vi "dfd_Render Real and Complex Roots+.vi"(0 "variable":string="z", 1 "alignment(left, top)":T3, 4 "display format":T2 items=["Separated Roots", "Combined Roots"], 5 "format coeffiecients":string, 6 "bracket":cluster{"left":string, "right":string}={"left"="(", "right"=")"}, 7 "fonts input":T5(array[cluster]), 8 "format control":T1={"display \"1\" when there are no roots"=TRUE, "bracket force to add"=FALSE}, 9 "origin":cluster{"x":i16, "y":i16}, 10 "Roots":cdb[](array[numeric]), 11 "picture in":picture) -> (2 "total rect":T4, 3 "picture out":picture)   [LabVIEW 2017, in "NI_DigFilter_Process.lvlib"]
uses:
  <vilib>/addons/Digital Filter Design/NI_DigFilter_Process.lvlib
  <vilib>/addons/Digital Filter Design/Render.llb/dfd_ZPK Display Format.ctl
  <vilib>/Analysis/NI_AALPro.lvlib
panel:
  in  "Tolerance for real roots":dbl
  in  "Tolerance for conjugate pair":dbl
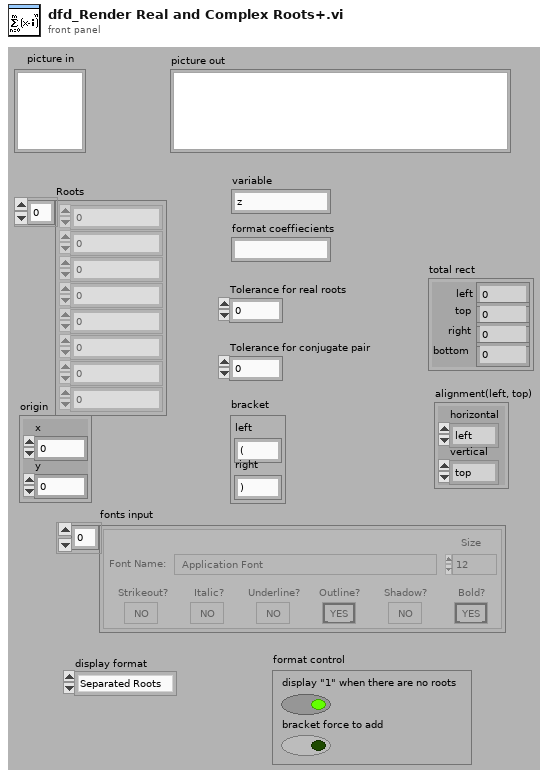
[diagram p1: front panel]
types:
  T1 = cluster{"display \"1\" when there are no roots":bool, "bracket force to add":bool}
  T2 = typedef "dfd_ZPK Display Format.ctl" = u16
  T3 = cluster{"horizontal":enum16{"left", "center", "right"}, "vertical":enum16{"top", "center", "bottom"}}
  T4 = cluster{"left":i16, "top":i16, "right":i16, "bottom":i16}
  T5 = cluster{"Font Name:":string, "Size":i16, "Strikeout?":bool, "Italic?":bool, "Underline?":bool, "Outline?":bool, "Shadow?":bool, "Bold?":bool}[]
  T6 = enum16{"User-specified Font", "Application Font", "System Font", "Dialog Font"}
  T7 = cluster{"Font Name:":string, "Size":i16, "Strikeout?":bool, "Italic?":bool, "Underline?":bool, "Outline?":bool, "Shadow?":bool, "Bold?":bool}
  T8 = typedef "imagedata.ctl" = cluster{"image type":i32, "image depth":i32, "image":u8[], "mask":u8[], "colors":u32[], "Rectangle":cluster{"left":i16, "top":i16, "right":i16, "bottom":i16}}
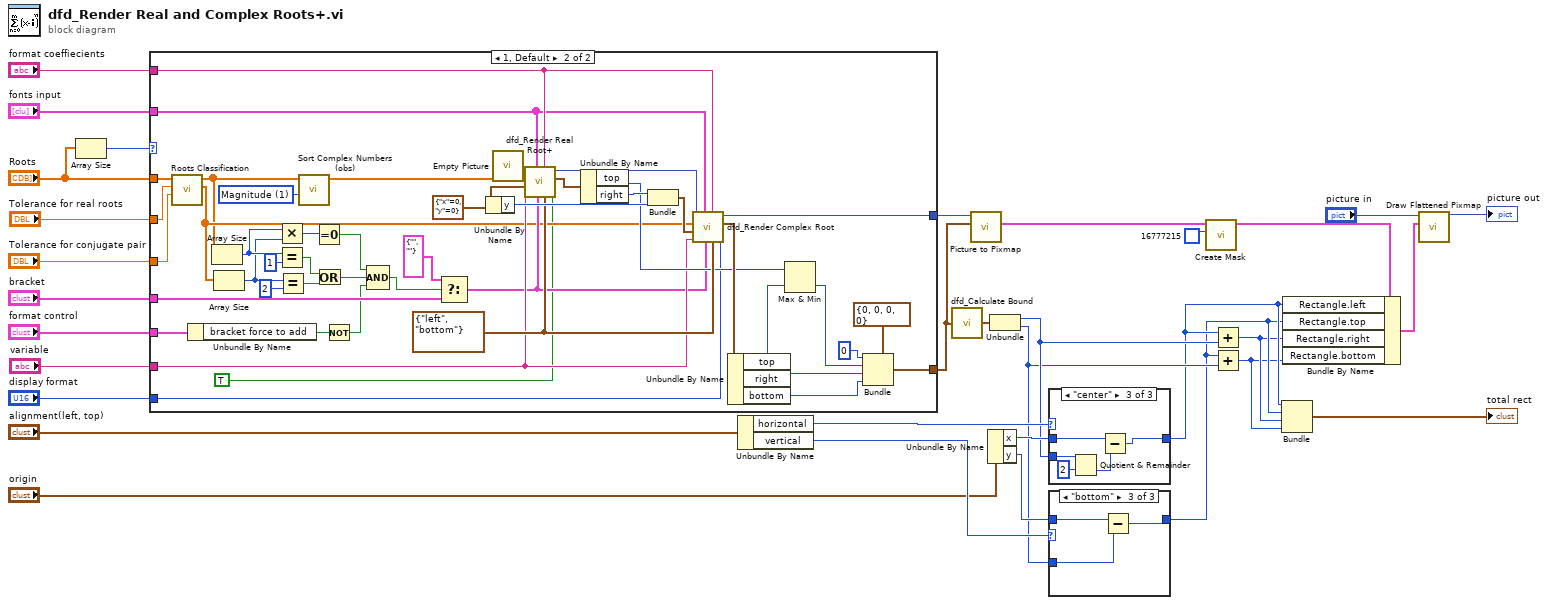
[diagram p0: block diagram]
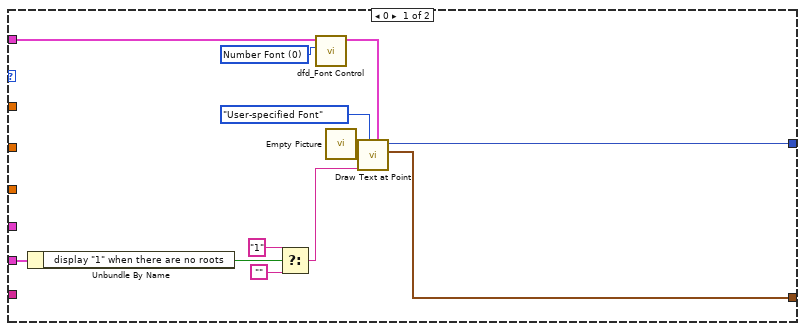
[diagram p2: hidden frame]
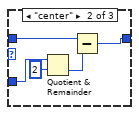
[diagram p4: hidden frame]
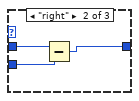
[diagram p6: hidden frame]
diagram:
  n1 = Array Size(array="Roots") -> (size(s)=w2:i32)
  n2 = case shown="1, Default" w2 {
    tunnel: "Tolerance for conjugate pair" -> [_ w90]
    tunnel: "Tolerance for real roots" -> [_ w89]
    tunnel: [w43 w83] -> w30
    tunnel: [w44 w77] -> w23
    tunnel: "format coeffiecients" -> [_ w69]
    tunnel: "fonts input" -> [w41 w68]
    tunnel: "display format" -> [_ w45]
    tunnel: "variable" -> [_ w66]
    tunnel: "Roots" -> [_ w65]
    tunnel: "bracket" -> [_ w62]
    tunnel: "format control" -> [w34 w49]
    frame 0 {
      w39 = u16 0 items=["Number Font", "Variable Font", "Script Font"] ("Tpye")
      n3 = Unbundle By Name(w34) -> ("display \"1\" when there are no roots"=w33:bool)
      n4 = Select(t="1" ("text"), s=w33, f="") -> (s? t:f=w36:string)
      n5 = call <vilib>:"dfd_Font Control.vi"("tpye"=w39, "fonts input"=w41) -> ("font output"=w40:T7)  [unwired: 9 out]
      n6 = call "Empty Picture"() -> ("empty picture"=w38:picture)
      n7 = call <vilib>:"Draw Text at Point.vi"("[user-specified font]"=w40, "desired font(Application)"=T6."User-specified Font", "text"=w36, "picture"=w38) -> ("text rect"=w44:T4, "new picture"=w43:picture)  [unwired: 5 in, 1 out]
    }
    frame 1, Default {
      w74 = cluster{"x":i16, "y":i16} {"x"=0, "y"=0} ("origin")
      w76 = T3 {"horizontal"=enum."left", "vertical"=enum."bottom"} ("alignment(left, top)")
      w88 = u16 1 items=["Real & Imaginary", "Magnitude"] ("method")
      n8 = call <vilib>:"Roots Classification.vi"("tolerance for conjugate pair"=w90, "tolerance for real roots"=w89, "Roots"=w65) -> ("Complex Pair Roots"=w60:cdb[], "Real Roots"=w58:dbl[])  [unwired: 7 out]
      n9 = Unbundle By Name(w49) -> ("bracket force to add"=w48:bool)
      n10 = Array Size(array=w58) -> (size(s)=w57:i32)
      n11 = Array Size(array=w60) -> (size(s)=w56:i32)
      n12 = Multiply(x=w57, y=w56) -> (x*y=w55:i32)
      n13 = Equal?(x=w57, y=1) -> (x = y?=w54:bool)
      n14 = Equal?(x=w56, y=2) -> (x = y?=w53:bool)
      n15 = call <vilib>:"Sort Complex Numbers (obs).vi"("method"=w88, "Complex Numbers"=w58) -> ("Sorted Complex Numbers"=w67:cdb[])  [unwired: 1 in, 8 out]
      n16 = Equal To 0?(x=w55) -> (x = 0?=w51:bool)
      n17 = Or(x=w54, y=w53) -> (x .or. y?=w52:bool)
      n18 = Not(x=w48) -> (.not. x?=w47:bool)
      n19 = Compound Arithmetic op=AND(w51, w52, w47) -> (w50:bool)
      n20 = Select(t=cluster{"left":string, "right":string} {"left"="", "right"=""} ("bracket"), s=w50, f=w62) -> (s? t:f=w61:cluster{"left":string, "right":string})
      n21 = Unbundle By Name(w74) -> ("y"=w78:i16)
      n22 = call "Empty Picture"() -> ("empty picture"=w73:picture)
      n23 = call <vilib>:"dfd_Render Real Root+.vi"("Negative Exponent?"=TRUE ("negative exponent? 2"), "alignment(left, top)"=w76, "format string"=w69, "bracket"=w61, "Fonts Input"=w68, "variable"=w66, "origin"=w74, "coefficients"=w67, "new picture"=w73) -> ("text rect"=w84:T4, "picture out"=w85:picture)  [unwired: 1 out]
      n24 = Unbundle By Name(w84) -> ("top"=w72:i16, "right"=w87:i16)
      n25 = Bundle("right"=w87, "y"=w78) -> (w86:cluster{"right":i16, "y":i16})  [unwired: 1 out]
      n26 = call <vilib>:"dfd_Render Complex Root.vi"("display format"=w45, "alignment(left, top)"=w76, "format string"=w69, "bracket"=w61, "Fonts Input"=w68, "variable"=w66, "origin"=w86, "complex numbers"=w60, "picture in"=w85) -> ("text rect"=w82:T4, "picture out"=w83:picture)  [unwired: 1 out]
      n27 = Unbundle By Name(w82) -> ("top"=w71:i16, "right"=w79:i16, "bottom"=w75:i16)
      n28 = Max & Min(x=w72, y=w71) -> (min(x,y)=w70:i16)  [unwired: 1 out]
      n29 = Bundle(cluster=T4 {"left"=0, "top"=0, "right"=0, "bottom"=0} ("total rect"), "left"=i16 0, "top"=w70, "right"=w79, "bottom"=w75) -> (w77:T4)
    }
  }
  n30 = Unbundle By Name("alignment(left, top)") -> ("horizontal"=w28:enum16{"left", "center", "right"}, "vertical"=w26:enum16{"top", "center", "bottom"})
  n31 = call <vilib>:"dfd_Calculate Bound.vi"("rect"=w23) -> ("Bounds"=w24:cluster{"Width":i16, "Height":i16})
  n32 = call <vilib>:"Picture to Pixmap.vi"("rect"=w23, "picture"=w30) -> ("image data"=w19:T8)  [unwired: 2 in, 7 out]
  n33 = Unbundle By Name("origin") -> ("x"=w27:i16, "y"=w25:i16)
  n34 = Unbundle(w24) -> ("Width"=w22:i16, "Height"=w21:i16)
  n35 = case shown="\"center\"" w28 {
    tunnel: w22 -> [_ w94 w97]
    tunnel: w27 -> [w91 w93 w96]
    tunnel: [w91 w92 w95] -> w17
    frame "left", Default {
    }
    frame "right" {
      n36 = Subtract(x=w93, y=w94) -> (x-y=w92:i16)
    }
    frame "center" {
      n37 = Quotient & Remainder(x=w97, y=i16 2) -> (floor(x/y)=w98:i16)  [unwired: 1 out]
      n38 = Subtract(x=w96, y=w98) -> (x-y=w95:i16)
    }
  }
  n39 = case shown="\"bottom\"" w26 {
    tunnel: w25 -> [w100 w103 w108]
    tunnel: [w100 w102 w106] -> w16
    tunnel: w21 -> [_ w101 w107]
    frame "top", Default {
    }
    frame "center" {
      n40 = Quotient & Remainder(x=w101, y=i16 2) -> (floor(x/y)=w104:i16)  [unwired: 1 out]
      n41 = Subtract(x=w103, y=w104) -> (x-y=w102:i16)
    }
    frame "bottom" {
      n42 = Subtract(x=w108, y=w107) -> (x-y=w106:i16)
    }
  }
  n43 = call <vilib>:"Create Mask.vi"("Mask Color (Black)"=u32 16777215, "image data"=w19) -> ("image data"=w18:T8)  [unwired: 2 in, 7 out]
  n44 = Add(x=w17, y=w22) -> (x+y=w15:i16)
  n45 = Add(x=w16, y=w21) -> (x+y=w14:i16)
  n46 = Bundle("x"=w17, "y"=w16, w15, w14) -> (→"total rect":cluster{"x":i16, "y":i16, i16, i16})  [unwired: 1 out]
  n47 = Bundle By Name(cluster=w18, "Rectangle.left"=w17, "Rectangle.top"=w16, "Rectangle.right"=w15, "Rectangle.bottom"=w14) -> (w29:T8)
  n48 = call <vilib>:"Draw Flattened Pixmap.vi"("image data"=w29, "picture"="picture in") -> ("new picture"=→"picture out":picture)  [unwired: 7 out]
